vi "Collection_Main.vi"() -> ()   [LabVIEW 2019]
uses:
  Control 1.ctl
  <vilib>/DAQmx/read.llb/DAQmx Read (Analog 1D Wfm NChan NSamp).vi
  <extravilib>/ChannelInstances/Stream-a[.](dbl)/Read With Abort.vi
  <extravilib>/ChannelInstances/Stream-a[.](dbl)/Write With Abort.vi
  <extravilib>/ChannelInstances/Stream-a[.](dbl)/EndpointRead.vi
  <extravilib>/ChannelInstances/Stream-a[.](dbl)/Endpoint.vi
  <vilib>/DAQmx/create/channels.llb/DAQmx Create Channel (AI-Voltage-Basic).vi
  <vilib>/DAQmx/configure/timing.llb/DAQmx Timing (Sample Clock).vi
  <vilib>/DAQmx/configure/trigger.llb/DAQmx Start Trigger (None).vi
  <vilib>/DAQmx/miscellaneous.llb/DAQmx Fill In Error Info.vi
  <extravilib>/ChannelInstances/Stream-a[.](dbl)/Instantiate.vi
  <extravilib>/ChannelInstances/Stream-a[.](dbl)/)Channel.vi
  <resource>/ChannelSupport/_ChannelSupport/WaitIfNeeded.vi
  <extravilib>/ChannelInstances/Stream-a[.](dbl).lvlib
panel:
  in  "Voltage Gain":string(combo)="1 X"
  in  "File Name":string="NAME_"
  in  "Vibrometer Settings":string(combo)="100 mm/s"
  out "Channel 1":dbl(graph)
  out "Channel 2":dbl(graph)
  out "Samples Ready":i32
  out "Number of Samples":i32
  out "Ready":bool
  in  "stop":bool
  in  "Save":bool
  in  "Post-Click Samples":i32=100
  in  "Collect":bool
  in  "Seconds to Capture":i32=2
  in  "Sampling Rate":dbl=10000.0 format="%#_13g"
  out "Realised Rate":dbl
  out "Live":waveform(dbl)[](graph)
  out "Loop Rate (Hz)":u32(knob) scale=0.0..5000.0
  # "SETTINGS"
  # "STATE"
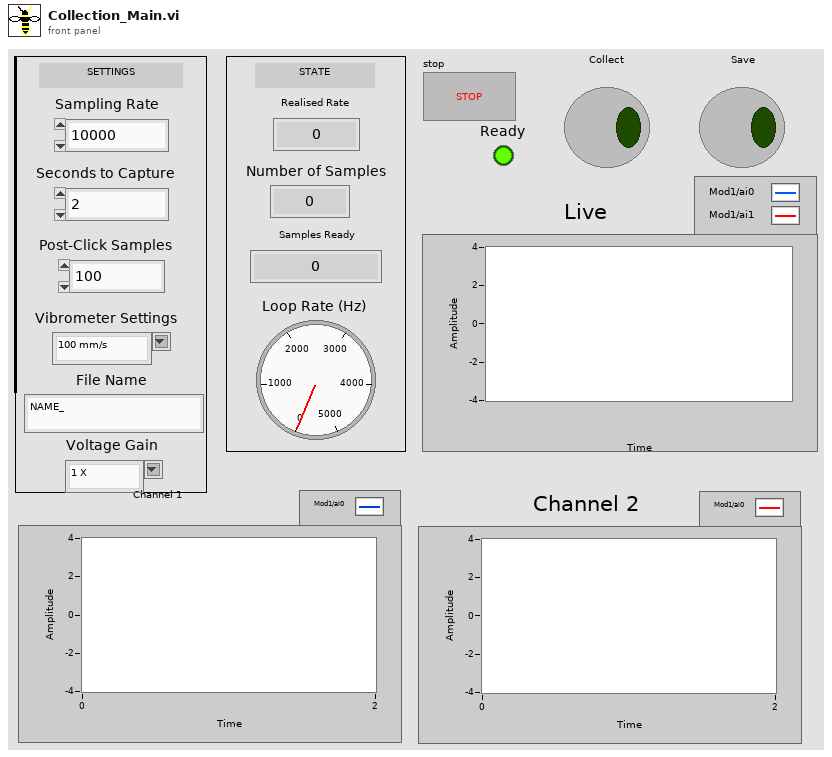
[diagram p1: front panel]
types:
  T1 = typedef "Control 1.ctl" = cluster{"Factor":dbl, "File name":string, "Data":dbl[][], "dT":dbl, "Voltage Gain":dbl}
  T2 = typedef "Stream-a[.](dbl).lvlib/)Channel.ctl" = refnum<queue>
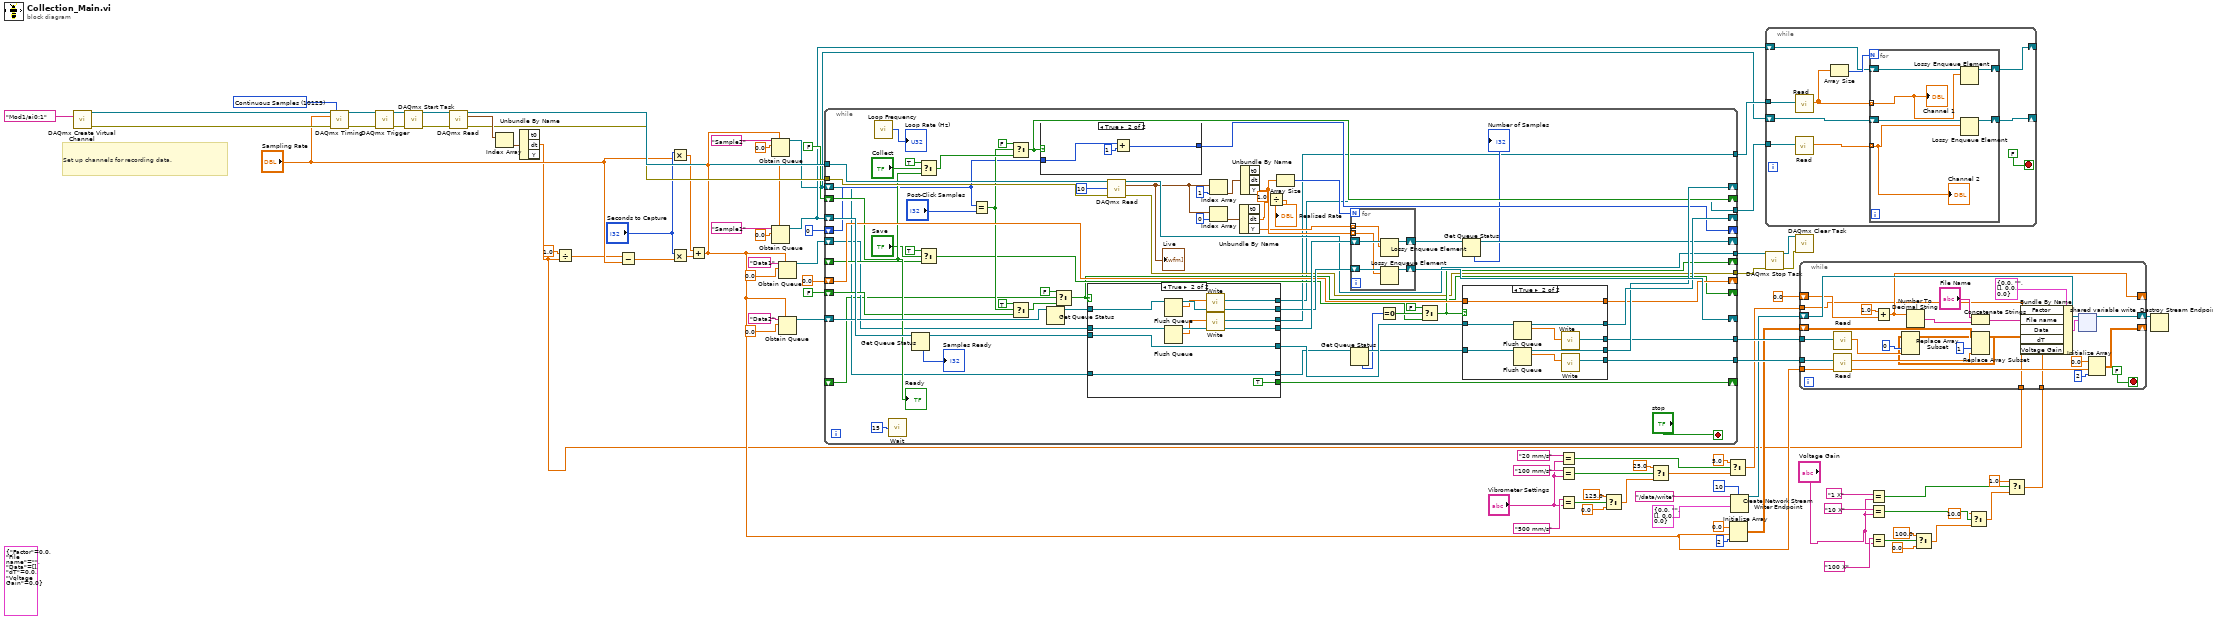
[diagram p0: block diagram]
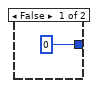
[diagram p2: hidden frame]
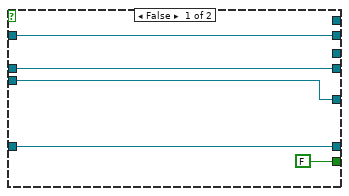
[diagram p4: hidden frame]
diagram:
  w69 = 10123 items=["Finite Samples"=10178, "Continuous Samples"=10123, "Hardware Timed Single Point"=12522] ("sample mode")
  (unwired) T1 {"Factor"=0.0, "File name"="", "Data"=[], "dT"=0.0, "Voltage Gain"=0.0}
  # "Set up channels for recording data."
  n1 = call-poly <vilib>:"DAQmx Create Virtual Channel.vi"("physical channels"=tag "Mod1/ai0:1") -> ("task out"=w76:refnum<k21>, "error out"=w75:errorcluster)  [unwired: 13 in]
  n2 = call-poly <vilib>:"DAQmx Timing.vi"("task/channels in"=w76, "sample mode"=w69, "rate"="Sampling Rate", "error in"=w75) -> ("task out"=w72:refnum<k21>, "error out"=w74:errorcluster)  [unwired: 10 in]
  n3 = call-poly <vilib>:"DAQmx Trigger.vi"("task/channels in"=w72, "error in"=w74) -> ("task out"=w71:refnum<k21>, "error out"=w73:errorcluster)  [unwired: 12 in]
  n4 = call <vilib>:"DAQmx Start Task.vi"("task/channels in"=w71, "error in"=w73) -> ("task out"=w68:refnum<k21>, "error out"=w67:errorcluster)  [unwired: 12 in]
  n5 = call-poly <vilib>:"DAQmx Read.vi"("task/channels in"=w68, "error in"=w67) -> ("task out"=w63:refnum<k21>, "data"=w65:waveform(dbl)[], "error out"=w62:errorcluster)  [unwired: 11 in]
  n6 = Index Array(array=w65) -> (element=w66:waveform(dbl))  [unwired: 1 in]
  n7 = Unbundle By Name(w66) -> ("dt"=w15:dbl)  [unwired: 2 out]
  n8 = Divide(x=1.0, y=w15) -> (x/y=w53:dbl)
  n9 = Subtract(x=w53, y="Sampling Rate") -> (x-y=w58:dbl)
  n10 = Multiply(x="Seconds to Capture", y="Sampling Rate") -> (x*y=w56:dbl)
  n11 = Multiply(x="Seconds to Capture", y=w58) -> (x*y=w55:dbl)
  n12 = Add(x=w56, y=w55) -> (x+y=w35:dbl)
  n13 = Obtain Queue(max queue size (-1, unlimited)=w35, name (unnamed)="Sample2", element data type=0.0) -> (queue out=w17:refnum<queue>)  [unwired: 2 in, 2 out]
  n14 = Obtain Queue(max queue size (-1, unlimited)=w35, name (unnamed)="Sample1", element data type=0.0) -> (queue out=w18:refnum<queue>)  [unwired: 2 in, 2 out]
  n15 = Obtain Queue(max queue size (-1, unlimited)=w35, name (unnamed)="Data1", element data type=0.0) -> (queue out=w61:refnum<queue>)  [unwired: 2 in, 2 out]
  n16 = Obtain Queue(max queue size (-1, unlimited)=w35, name (unnamed)="Data2", element data type=0.0) -> (queue out=w60:refnum<queue>)  [unwired: 2 in, 2 out]
  n17 = while {
    tunnel: w63 -> [w146]
    tunnel: w62 -> [w145]
    shift-right: [w104] -> _
    shift-left: w61 -> [w100]
    shift-right: [w142] -> _
    shift-left: w60 -> [w137]
    shift-right: [w134] -> _
    shift-left: w18 -> [w139]
    shift-right: [w132] -> _
    shift-left: w17 -> [w102]
    shift-right: [w130] -> _
    shift-left: 0.0 -> [w131]
    shift-right: [w117] -> _
    shift-left: FALSE ("t") -> [w127]
    shift-right: [w98] -> _
    shift-left: FALSE -> [w120]
    shift-right: [w111] -> _
    shift-left: _ -> [w109]
    tunnel: [w108] -> w50
    tunnel: [w107] -> w49
    shift-right: [w125] -> _
    shift-left: 0 -> [w105]
    shift-right: [w94] -> _
    shift-left: _ -> [w95]
    tunnel: [w93] -> w45
    tunnel: [w92] -> w44
    tunnel: [w91] -> w20
    tunnel: [w90] -> w19
    stop <- "stop" stop-if-true
    n18 = call "Loop Frequency.vi"() -> ("Loop Rate (Hz)"=→"Loop Rate (Hz)":u32)
    n19 = call "Wait"("Count(uSec)"=u32 15) -> ()  [unwired: 1 out]
    n20 = Get Queue Status(queue=w139) -> (queue out=w101:refnum<queue>, # elements in queue=→"Samples Ready":i32)  [unwired: 2 in, 6 out]
    n21 = Select(t=TRUE, s="Collect", f=w127) -> (s? t:f=w126:bool)
    n22 = Select(t=TRUE, s="Save", f=w109) -> (s? t:f=w112:bool)
    n23 = Equal?(x=w105, y="Post-Click Samples") -> (x = y?=w122:bool)
    n24 = Select(t=FALSE, s=w122, f=w126) -> (s? t:f=w117:bool)
    n25 = Select(t=TRUE, s=w122, f=w120) -> (s? t:f=w119:bool)
    n26 = case shown="True" w117 {
      tunnel: w105 -> [_ w156]
      tunnel: [0 w155] -> w125
      frame False {
      }
      frame True {
        n27 = Add(x=w156, y=1) -> (x+y=w155:i32)
      }
    }
    n28 = Get Queue Status(queue=w137) -> (queue out=w97:refnum<queue>)  [unwired: 2 in, 7 out]
    n29 = Select(t=FALSE, s=w95, f=w119) -> (s? t:f=w98:bool)
    n30 = case shown="True" w98 {
      tunnel: w101 -> [w172 w178]
      tunnel: [w172 w178] -> w135
      tunnel: w102 -> [w170 w177]
      tunnel: [w170 w177] -> w133
      tunnel: w100 -> [w173 w184]
      tunnel: [w173 w182] -> w138
      tunnel: w97 -> [w171 w183]
      tunnel: [w171 w181] -> w136
      tunnel: [FALSE TRUE] -> w94
      tunnel: [_ w175] -> w91
      tunnel: [_ w174] -> w90
      frame False {
      }
      frame True {
        n31 = Flush Queue(queue=w183) -> (queue out=w181:refnum<queue>, remaining elements=w176:dbl[])  [unwired: 1 in, 1 out]
        n32 = Flush Queue(queue=w184) -> (queue out=w182:refnum<queue>, remaining elements=w180:dbl[])  [unwired: 1 in, 1 out]
        n33 = call <extravilib>:"Write.vi"("element"=w176) -> ("channel"=w174:T2)  [unwired: 8 in, 2 out]
        n34 = call <extravilib>:"Write.vi"("element"=w180) -> ("channel"=w175:T2)  [unwired: 8 in, 2 out]
      }
    }
    n35 = call-poly <vilib>:"DAQmx Read.vi"("task/channels in"=w146, "number of samples per channel"=10, "error in"=w145) -> ("task out"=w108:refnum<k21>, "data"=w86:waveform(dbl)[], "error out"=w107:errorcluster)  [unwired: 10 in]
    "Live" <- w86
    n36 = Index Array(array=w86, index=1) -> (element=w147:waveform(dbl))
    n37 = Index Array(array=w86, index=0) -> (element=w149:waveform(dbl))
    n38 = Unbundle By Name(w149) -> ("dt"=w88:dbl, "Y"=w140:dbl[])  [unwired: 1 out]
    n39 = Unbundle By Name(w147) -> ("Y"=w141:dbl[])  [unwired: 2 out]
    n40 = Divide(x=1.0, y=w88) -> (x/y=→"Realised Rate":dbl)
    n41 = Array Size(array=w141) -> (size(s)=w144:i32)
    n42 = for {
      N: w144 -> [_]
      shift-right: [w188] -> w143
      shift-left: w138 -> [w190]
      shift-right: [w187] -> w142
      shift-left: w136 -> [w189]
      tunnel: w141 -> [w186] mode=indexing
      tunnel: w140 -> [w185] mode=indexing
      n43 = Lossy Enqueue Element(queue=w190, element=w185) -> (queue out=w188:refnum<queue>)  [unwired: 1 in, 3 out]
      n44 = Lossy Enqueue Element(queue=w189, element=w186) -> (queue out=w187:refnum<queue>)  [unwired: 1 in, 3 out]
    }
    n45 = Get Queue Status(queue=w133) -> (queue out=w114:refnum<queue>, # elements in queue=w96:i32)  [unwired: 2 in, 6 out]
    n46 = Equal To 0?(x=w96) -> (x = 0?=w113:bool)
    n47 = Select(t=FALSE, s=w113, f=w112) -> (s? t:f=w111:bool)
    n48 = Get Queue Status(queue=w143) -> (queue out=w104:refnum<queue>, # elements in queue=→"Number of Samples":i32)  [unwired: 2 in, 6 out]
    n49 = case shown="True" w111 {
      tunnel: w135 -> [w159 w168]
      tunnel: [w159 w166] -> w134
      tunnel: w114 -> [w158 w167]
      tunnel: [w158 w165] -> w132
      tunnel: w131 -> [w157 w164]
      tunnel: [w157 w164] -> w130
      tunnel: [_ w163] -> w93
      tunnel: [_ w162] -> w92
      frame False {
      }
      frame True {
        n50 = Flush Queue(queue=w168) -> (queue out=w166:refnum<queue>, remaining elements=w160:dbl[])  [unwired: 1 in, 1 out]
        n51 = Flush Queue(queue=w167) -> (queue out=w165:refnum<queue>, remaining elements=w161:dbl[])  [unwired: 1 in, 1 out]
        n52 = call <extravilib>:"Write.vi"("element"=w160) -> ("channel"=w163:T2)  [unwired: 8 in, 2 out]
        n53 = call <extravilib>:"Write.vi"("element"=w161) -> ("channel"=w162:T2)  [unwired: 8 in, 2 out]
      }
    }
    "Ready" <- w127
  }
  n54 = Equal?(x="20 mm/s", y="Vibrometer Settings") -> (x = y?=w26:bool)
  n55 = Equal?(x="100 mm/s", y="Vibrometer Settings") -> (x = y?=w29:bool)
  n56 = Equal?(x="500 mm/s", y="Vibrometer Settings") -> (x = y?=w32:bool)
  n57 = Select(t=125.0, s=w32, f=0.0) -> (s? t:f=w30:dbl)
  n58 = Select(t=25.0, s=w29, f=w30) -> (s? t:f=w25:dbl)
  n59 = Select(t=5.0, s=w26, f=w25) -> (s? t:f=w21:dbl)
  n60 = Initialize Array(0.0 ("element"), w35, 2 ("dimension size")) -> (w41:dbl[][])
  n61 = Create Network Stream Writer Endpoint(7:10 ("writer buffer size"), 9:T1 {"Factor"=0.0, "File name"="", "Data"=[], "dT"=0.0, "Voltage Gain"=0.0}, 11:"/data/write" ("reader url")) -> (3:w37:refnum<k21>)  [unwired: 4 in, 1 out]
  n62 = while {
    tunnel: w20 -> [w200]
    tunnel: w19 -> [w199]
    shift-right: [w194] -> _
    shift-left: w18 -> [w196]
    shift-right: [w193] -> _
    shift-left: w17 -> [w195]
    stop <- FALSE stop-if-true
    n63 = call <extravilib>:"Read.vi"("channel"=w199) -> ("element"=w191:dbl[])  [unwired: 6 in, 4 out]
    n64 = call <extravilib>:"Read.vi"("channel"=w200) -> ("element"=w198:dbl[])  [unwired: 6 in, 4 out]
    n65 = Array Size(array=w198) -> (size(s)=w197:i32)
    n66 = for {
      N: w197 -> [_]
      shift-right: [w203] -> w194
      shift-left: w196 -> [w204]
      shift-right: [w205] -> w193
      shift-left: w195 -> [w206]
      tunnel: w191 -> [w202] mode=indexing
      tunnel: w198 -> [w201] mode=indexing
      n67 = Lossy Enqueue Element(queue=w204, element=w201) -> (queue out=w203:refnum<queue>)  [unwired: 1 in, 3 out]
      n68 = Lossy Enqueue Element(queue=w206, element=w202) -> (queue out=w205:refnum<queue>)  [unwired: 1 in, 3 out]
      "Channel 1" <- w201
      "Channel 2" <- w202
    }
  }
  n69 = call <vilib>:"DAQmx Stop Task.vi"("task/channels in"=w50, "error in"=w49) -> ("task out"=w48:refnum<k21>, "error out"=w47:errorcluster)  [unwired: 12 in]
  n70 = call <vilib>:"DAQmx Clear Task.vi"("task in"=w48, "error in"=w47) -> ()  [unwired: 13 in, 1 out]
  n71 = Equal?(x="1 X", y="Voltage Gain") -> (x = y?=w4:bool)
  n72 = Equal?(x="10 X", y="Voltage Gain") -> (x = y?=w7:bool)
  n73 = Equal?(x="100 X", y="Voltage Gain") -> (x = y?=w13:bool)
  n74 = Select(t=100.0, s=w13, f=0.0) -> (s? t:f=w8:dbl)
  n75 = Select(t=10.0, s=w7, f=w8) -> (s? t:f=w5:dbl)
  n76 = Select(t=1.0, s=w4, f=w5) -> (s? t:f=w2:dbl)
  n77 = while {
    tunnel: w45 -> [w222]
    tunnel: w44 -> [w220]
    shift-right: [w218] -> _
    shift-left: w41 -> [w210]
    shift-right: [w223] -> w36
    shift-left: w37 -> [w217]
    tunnel: w35 -> [w215]
    shift-right: [w213] -> _
    shift-left: 0.0 -> [w214]
    tunnel: w21 -> [w212]
    tunnel: w15 -> [w211]
    tunnel: w2 -> [w207]
    stop <- FALSE stop-if-true
    n78 = call <extravilib>:"Read.vi"("channel"=w222) -> ("element"=w221:dbl[])  [unwired: 6 in, 4 out]
    n79 = call <extravilib>:"Read.vi"("channel"=w220) -> ("element"=w219:dbl[])  [unwired: 6 in, 4 out]
    n80 = Add(x=1.0, y=w214) -> (x+y=w213:dbl)
    n81 = Number To Decimal String(number=w213) -> (decimal integer string=w227:string)  [unwired: 1 in]
    n82 = Concatenate Strings("File Name", w227) -> (w225:string)
    n83 = Replace Array Subset(array=w210, new element=w219, index (col)=1 ("disabled index (col)")) -> (w209:dbl[][])  [unwired: 1 in]
    n84 = Replace Array Subset(array=w209, new element=w221, index (col)=0 ("disabled index (col)")) -> (w208:dbl[][])  [unwired: 1 in]
    n85 = Bundle By Name(cluster=T1 {"Factor"=0.0, "File name"="", "Data"=[], "dT"=0.0, "Voltage Gain"=0.0}, "Factor"=w212, "File name"=w225, "Data"=w208, "dT"=w211, "Voltage Gain"=w207) -> (w224:T1)
    n86 = shared-variable-write(w217, w224) -> (w223:refnum<k21>)  [unwired: 2 in, 2 out]
    n87 = Initialize Array(0.0 ("element"), w215, 2 ("dimension size")) -> (w218:dbl[][])
  }
  n88 = Destroy Stream Endpoint(11:w36) -> ()  [unwired: 1 in, 1 out]
